vi "Main.vi"(11 "Module Admin":refnum<class "Delacor_lib_QMH_Module Admin.lvclass">) -> ()   [LabVIEW 2022 SP3, in "Event Manager.lvlib"]
doc: "This template is based from the Queued Message Handler design pattern and the Queued Message Handler Project Template that ships with LabVIEW 2014.\n\nThe main difference is that the Queue is private to this module and communication between modules is done via Broadcast and Request events.\n\nRequest events are wrapped via public API methods and are handled in the Event handler loop in this VI.\nAny module can register for Broadcast events sent by this module.\n\nThe Event Handling Loop generates messages based on user interface actions.\n\nThe Message Handling Loop processes messages generated by the Event Handling Loop, or by other messages. The messages are string values, so new messages can be added easily to the Message Cases case structure in the Message Handling Loop. Each message cluster can also provide an optional value for Message Data, which is a variant that can be converted to whatever message-specific data is required.\n____\nHAMPEL SOFTWARE ENGINEERING v2.6.0 (2023-12-19 10:54)"
uses:
  Event Manager.lvlib
  <vilib>/Delacor/Delacor QMH/Libraries/Module Admin_class/Delacor_lib_QMH_Module Admin.lvclass
  Libraries/hse-libraries/Source/hse-dqmh/Dynamic Requesters/Singleton/Status Updated Argument--cluster.ctl
  Libraries/hse-libraries/Source/hse-dqmh/Dynamic Requesters/Singleton/Error Reported Argument--cluster.ctl
  Libraries/hse-libraries/Source/hse-dqmh/Controls/System Message Argument--cluster.ctl
  Libraries/hse-libraries/Source/hse-dqmh/Controls/System Message Source.ctl
  Module Data--cluster.ctl
  Stop Argument--cluster.ctl
  <vilib>/Delacor/Delacor QMH/Libraries/Message Queue_class/Delacor_lib_QMH_Message Queue.lvclass/Delacor_lib_QMH_Message Queue.ctl
  <vilib>/Delacor/Delacor QMH/Libraries/Module Admin_class/Delacor_lib_QMH_Module Admin.lvclass/Delacor_lib_QMH_Module Admin.ctl
  Configure Argument--cluster.ctl
  Prepare Argument--cluster.ctl
  Set Modules Argument--cluster.ctl
  Set Modules (Reply Payload)--cluster.ctl
  <vilib>/Hampel Software Engineering/HSE Logger/LogRecord/LogRecord.lvclass/LogRecord.ctl
  Request UI Display Argument--cluster.ctl
  Libraries/hse-libraries/Source/hse-dqmh/Controls/Module Display Scenarios.ctl
  Request UI Display (Reply Payload)--cluster.ctl
  <vilib>/Utility/miscctls.llb/LVPointTypeDef.ctl
  <vilib>/Hampel Software Engineering/HSE Logger/LogRecord/LogRecord.lvclass
  <vilib>/Delacor/Delacor QMH/Libraries/Message Queue_class/Delacor_lib_QMH_Enqueue Message (Single).vi
  <vilib>/Delacor/Delacor QMH/Libraries/Module Admin_class/Delacor_lib_QMH_Get External Launch.vi
  <vilib>/Utility/error.llb/Error Cluster From Error Code.vi
  <vilib>/ErrorRing/Error Ring.xnode
  <vilib>/Delacor/Delacor QMH/Libraries/Message Queue_class/Delacor_lib_QMH_Message Queue.lvclass
  Libraries/hse-libraries/Source/hse-configuration/config-ini/config-ini.lvclass
  <vilib>/Hampel Software Engineering/HSE Logger/hse-logger.lvlib
  Libraries/hse-libraries/Source/hse-dqmh/hse-dqmh-dynamicrequesters.lvlib
  Libraries/hse-libraries/Source/hse-dqmh/hse-dqmh.lvlib
  Libraries/hse-libraries/Source/hse-misc/hse-misc.lvlib
panel:
  out "max rows":i32
  out "Status Bar":string
  in  "Event Log":i32(listbox)=-1
  out "error out":errorcluster
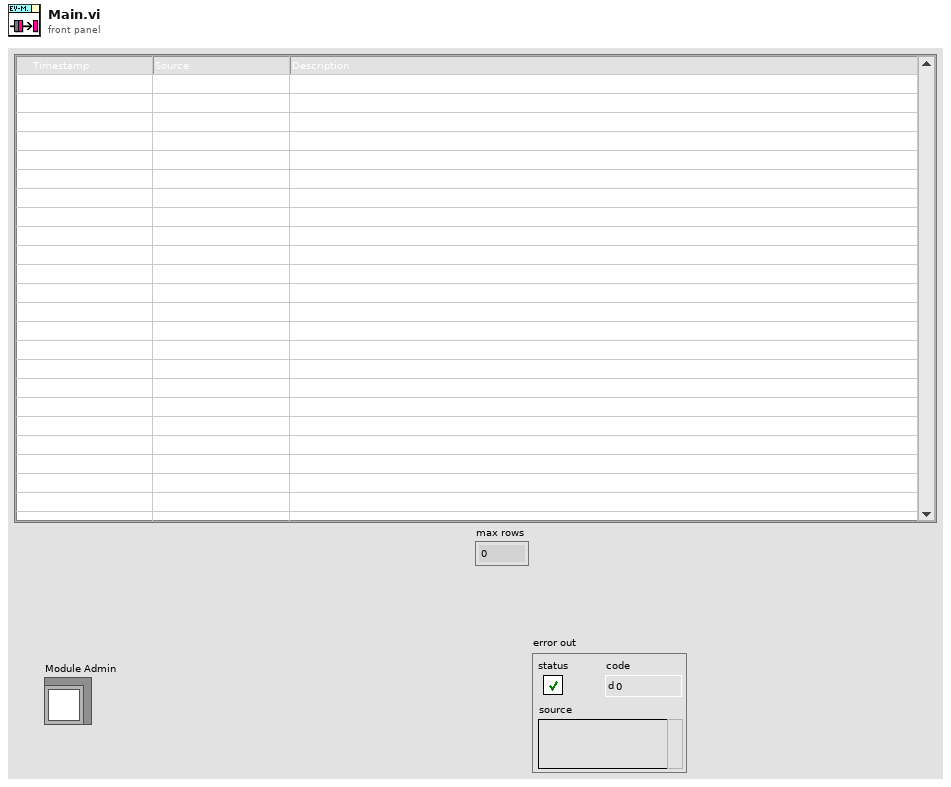
[diagram p1: front panel]
types:
  T1 = typedef "Event Manager.lvlib/Request Events--cluster.ctl" = cluster{"Stop Module":refnum<user-event>, "Show Panel":refnum<user-event>, "Hide Panel":refnum<user-event>, "Get Module Execution Status":refnum<user-event>, "Show Diagram":refnum<user-event>, "Configure":refnum<user-event>, "Prepare":refnum<user-event>, "Register for module events":refnum<user-event>, "Set Modules":refnum<user-event>, "Request UI Display":refnum<user-event>}
  T2 = typedef "Event Manager.lvlib/Module Data--cluster.ctl" = cluster{"Module Paths":path[]}
  T3 = enum32{"Invalid", "Standard", "Closed", "Hidden", "Minimized", "Maximized"}
  T4 = enum32{"invalid lock state", "Not Locked", "Locked (No Password)", "Password-protected"}
  T5 = typedef "Event Manager.lvlib/Stop Argument--cluster.ctl" = cluster{"Origin":string, "Exit via Stop Module Req?":bool, "Wait for Module to stop?":bool}
  T6 = typedef "Event Manager.lvlib/Configure Argument--cluster.ctl" = cluster{"Boolean":bool}
  T7 = typedef "Event Manager.lvlib/Prepare Argument--cluster.ctl" = cluster{"Boolean":bool}
  T8 = typedef "Event Manager.lvlib/Set Modules Argument--cluster.ctl" = cluster{"Module Paths":path[], "Wait Notifier":refnum<notifier>, "wait for reply":bool}
  T9 = typedef "Event Manager.lvlib/Request UI Display Argument--cluster.ctl" = cluster{"Scenario":T10, "Wait Notifier":refnum<notifier>, "wait for reply":bool}
  T10 = typedef "hse-dqmh.lvlib/Module Display Scenarios.ctl" = enum16{"Stand-Alone", "Managed"}
  T11 = typedef "LVPointTypeDef.ctl" = cluster{"Horizontal":i16, "Vertical":i16}
  T12 = typedef "Event Manager.lvlib/Request UI Display (Reply Payload)--cluster.ctl" = cluster{"Accept?":bool, "error":errorcluster}
  T13 = typedef "Event Manager.lvlib/Set Modules (Reply Payload)--cluster.ctl" = cluster{"Set Modules_error":errorcluster}
  T14 = typedef "LVRectTypeDef.ctl" = cluster{"Left":i16, "Top":i16, "Right":i16, "Bottom":i16}
  T15 = typedef "hse-logger.lvlib/LogLevel.ctl" = enum16{"DEBUG", "INFO", "WARNING", "ERROR", "CRITICAL"}
  T16 = typedef "hse-dqmh.lvlib/System Message Source.ctl" = enum16{"module", "application", "network"}
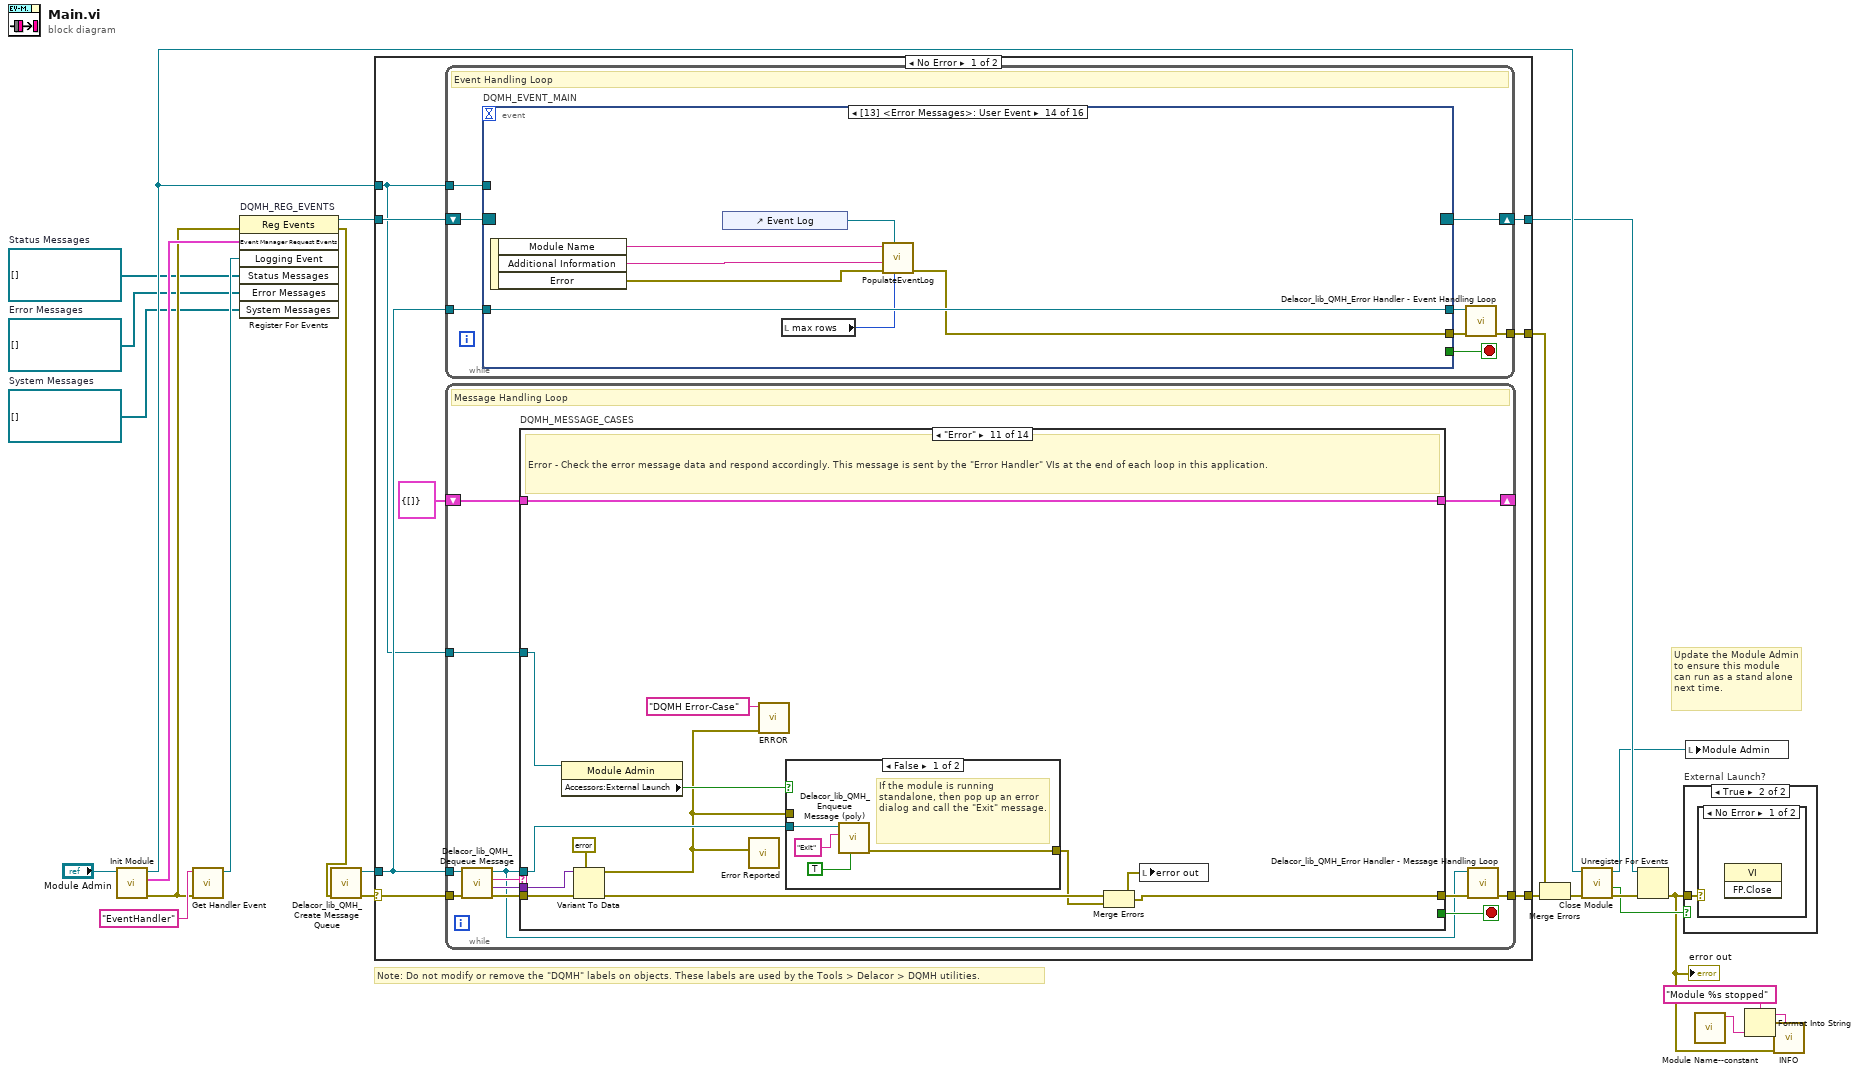
[diagram p0: block diagram]
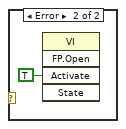
[diagram p3: hidden frame]
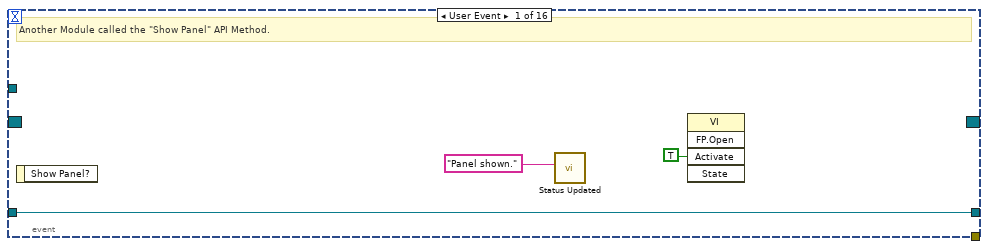
[diagram p4: hidden frame]
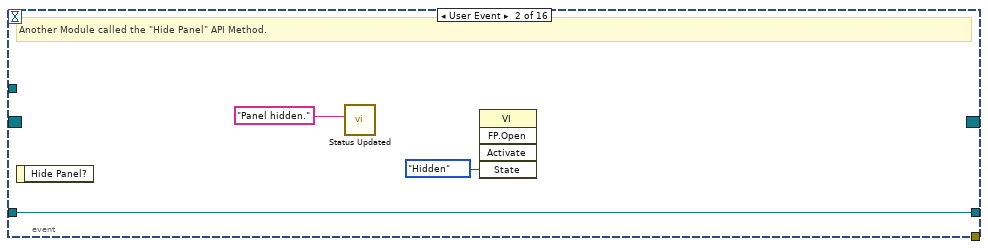
[diagram p5: hidden frame]
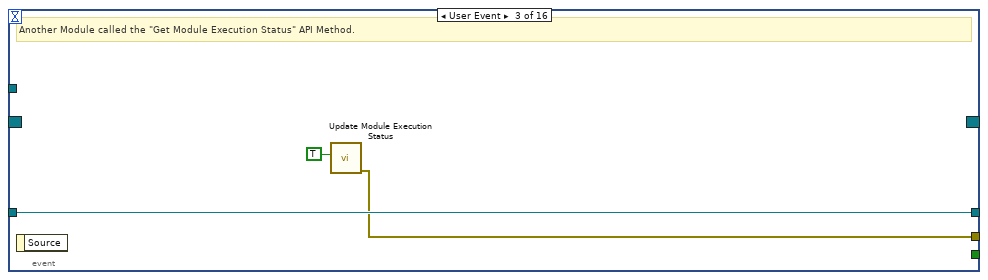
[diagram p6: hidden frame]
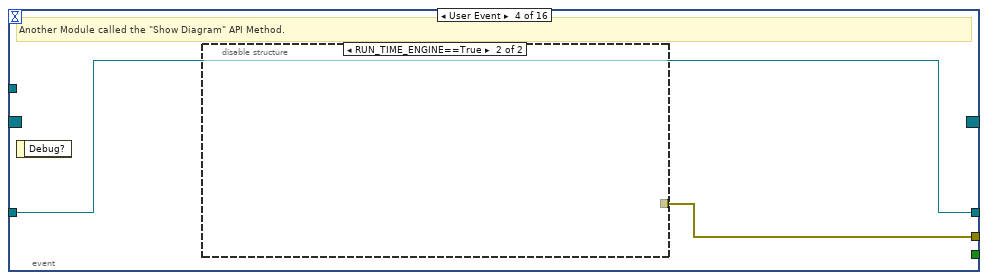
[diagram p7: hidden frame]
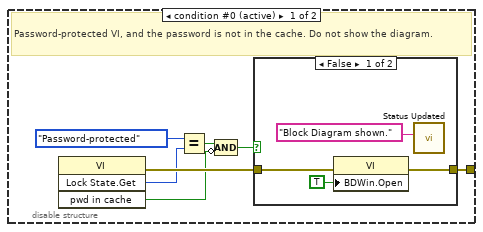
[diagram p8: hidden frame]
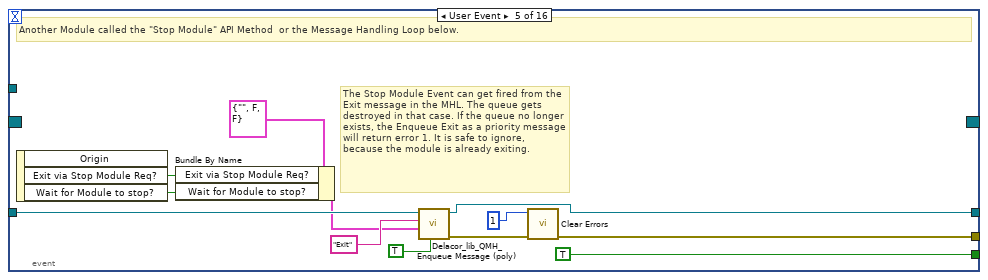
[diagram p10: hidden frame]
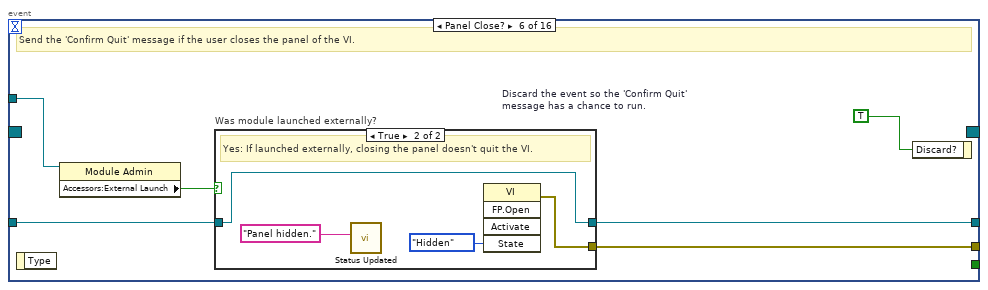
[diagram p11: hidden frame]
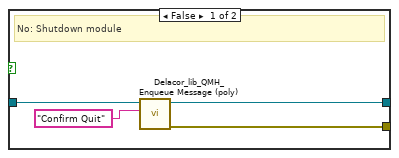
[diagram p12: hidden frame]
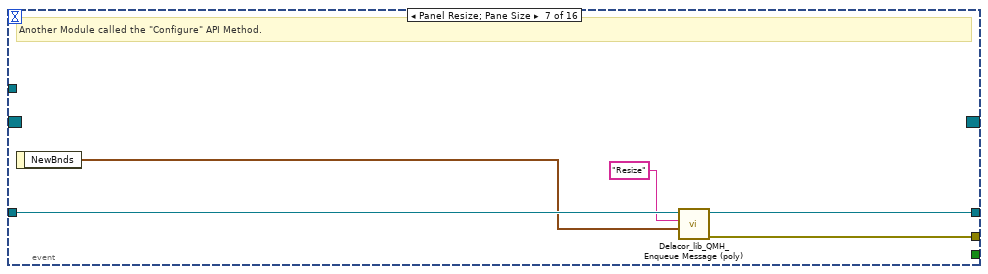
[diagram p13: hidden frame]
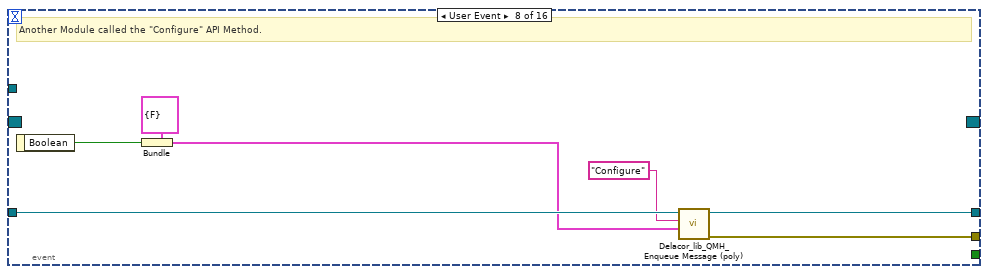
[diagram p14: hidden frame]
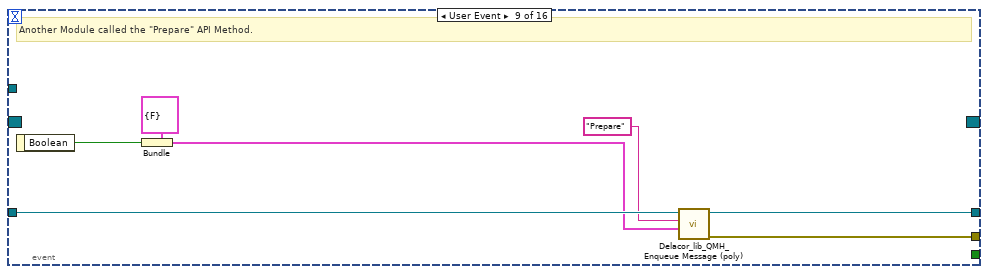
[diagram p15: hidden frame]
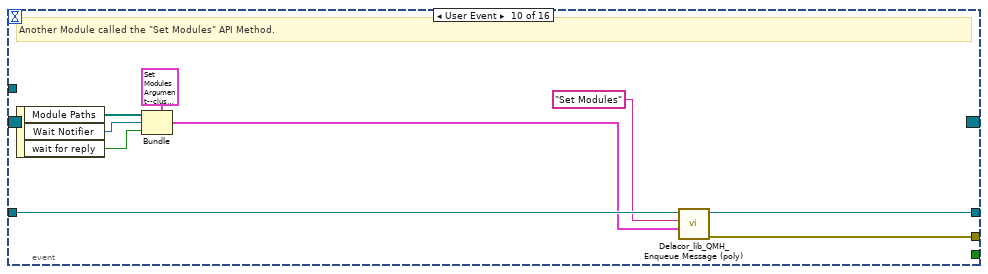
[diagram p16: hidden frame]
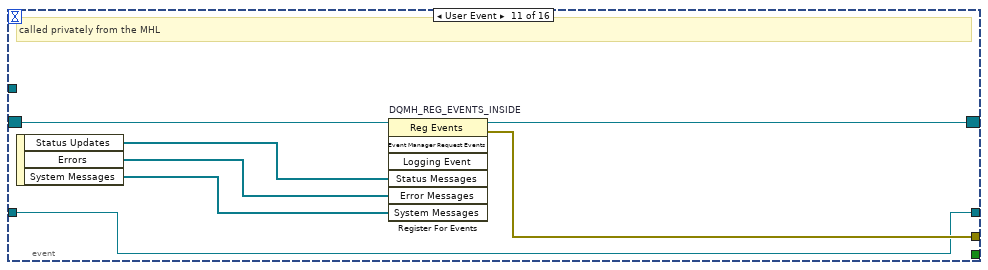
[diagram p17: hidden frame]
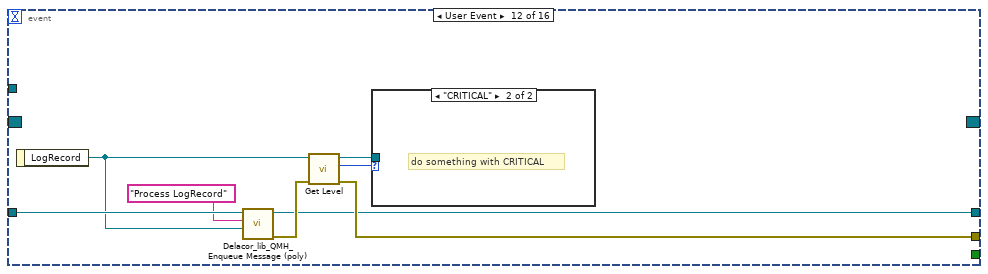
[diagram p18: hidden frame]
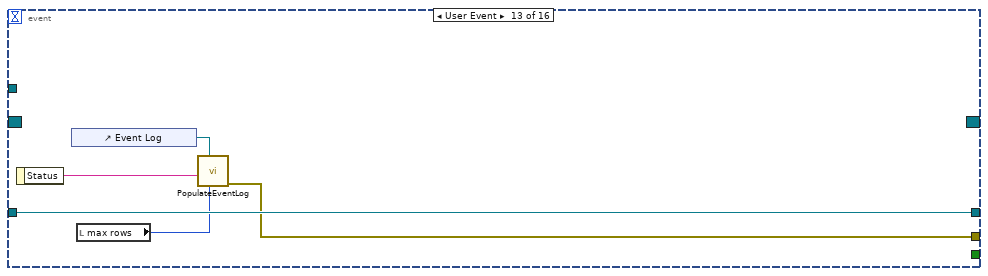
[diagram p20: hidden frame]
diagram:
  w1 = refnum<user-event>[] []  # System Messages
  w2 = refnum<user-event>[] []  # Error Messages
  w3 = refnum<user-event>[] []  # Status Messages
  # "Note: Do not modify or remove the \"DQMH\" labels on objects. These labels are used by the Tools > Delacor > DQMH utilities."
  # "Update the Module Admin to ensure this module can run as a stand alone next time."
  n1 = call "Init Module.vi"("Singleton Module Admin in"="Module Admin") -> ("error out"=w5:errorcluster, "Event Manager Request Events"=w20:T1, "Singleton Module Admin out"=w24:refnum<class "Delacor_lib_QMH_Module Admin.lvclass">)  [unwired: 8 in]
  n2 = call <vilib>:"Get Handler Event.vi"("error in"=w5, "Name"="EventHandler") -> ("Logging Event"=w11:refnum<user-event>)  [unwired: 8 in, 1 out]
  n3 = register-events "DQMH_REG_EVENTS"(error in=w5, w20, w11, w3, w2, w1) -> (reference out=w21:refnum<event-registration>, error out=w4:errorcluster)  [unwired: 1 in]
  n4 = call <vilib>:"Delacor_lib_QMH_Create Message Queue.vi"("error in"=w4) -> ("error out"=w12:errorcluster, "Message Queue"=w19:refnum<class "Delacor_lib_QMH_Message Queue.lvclass">)  [unwired: 9 in]
  n5 = case shown="No Error" w12 {
    selector: w12 -> [w26 w372]
    tunnel: [w32 w372] -> w23
    tunnel: [w31 w377] -> w22
    tunnel: w21 -> [w29 w377]
    tunnel: w19 -> [w28 w369]
    tunnel: [w27 _] -> w15
    tunnel: w24 -> [w25 w373]
    frame No Error {
      n6 = while {
        tunnel: w28 -> [w40]
        shift-right: [w38] -> w31
        shift-left: w29 -> [w39]
        tunnel: [w34] -> w27
        tunnel: w25 -> [w33]
        stop <- w36 stop-if-true
        # "Event Handling Loop"
        n7 = event "DQMH_EVENT_MAIN" shown="[13] <Error Messages>: User Event" {
          selector: w39 -> [_ _ _ _ _ _ _ _ _ _ w124 _ _ _ _ _]
          dyn-events: [_ _ _ _ _ _ _ _ _ _ w123 _ _ _ _ _] -> w38
          timeout: _ -> [_ _ _ _ _ _ _ _ _ _ _ _ _ _ _ _]
          tunnel: [_ _ _ _ TRUE ("Discard?") _ _ _ _ _ _ _ _ _ _ _] -> w36
          tunnel: w40 -> [w43 w46 w49 w50 w73 w80 w94 w101 w108 w117 w118 w130 w137 w144 w155 w165]
          tunnel: [_ _ w48 w51 w68 w79 w91 w95 w102 w109 w119 w132 w134 w142 w156 w157] -> w37
          tunnel: [w43 w46 w49 w50 w72 w78 w93 w100 w107 w116 w118 w129 w137 w144 w155 w164] -> w35
          tunnel: w33 -> [_ _ _ _ _ w77 _ _ _ _ _ _ _ _ _ _]
          event User Event {
            # "Another Module called the \"Show Panel\" API Method."
            n8 = event-data() -> ()  [unwired: 1 in, 1 out]
            n9 = call "Status Updated.vi"("Status"="Panel shown." ("format string")) -> ()  [unwired: 10 in, 1 out]
            n10 = invoke class="VI" method="FP.Open"("Activate"=TRUE ("Activate?")) -> ()  [unwired: 4 in, 5 out]
          }
          event User Event {
            # "Another Module called the \"Hide Panel\" API Method."
            n11 = event-data() -> ()  [unwired: 1 in, 1 out]
            n12 = call "Status Updated.vi"("Status"="Panel hidden." ("format string")) -> ()  [unwired: 10 in, 1 out]
            n13 = invoke class="VI" method="FP.Open"("State"=T3."Hidden") -> ()  [unwired: 4 in, 5 out]
          }
          event User Event {
            # "Another Module called the \"Get Module Execution Status\" API Method."
            n14 = event-data() -> ()  [unwired: 1 in, 1 out]
            n15 = call "Update Module Execution Status.vi"("Running?"=TRUE) -> ("error out"=w48:errorcluster)  [unwired: 10 in]
          }
          event User Event {
            # "Another Module called the \"Show Diagram\" API Method."
            n16 = event-data() -> ()  [unwired: 1 in, 1 out]
            n17 = disable-structure shown="RUN_TIME_ENGINE==True" {
              disable-tunnel: [w58 _] -> w51
              frame condition #0 (active) {
                # "Password-protected VI, and the password is not in the cache. Do not show the diagram."
                n18 = invoke class="VI" method="Lock State.Get"() -> (error out=w57:errorcluster, "Get Lock State"=w56:T4, "pwd in cache"=w53:bool)  [unwired: 4 in, 1 out]
                n19 = Equal?(x=T4."Password-protected", y=w56) -> (x = y?=w54:bool)
                n20 = Compound Arithmetic op=AND(w54, invert w53) -> (w52:bool)
                n21 = case shown="False" w52 {
                  tunnel: [w61 w63] -> w58
                  tunnel: w57 -> [w59 w63]
                  frame False {
                    n22 = property class="VI"(error in=w59, "BDWin.Open"=TRUE ("Block Diagram Window:Open")) -> (error out=w61:errorcluster)  [unwired: 1 in, 1 out]
                    n23 = call "Status Updated.vi"("Status"="Block Diagram shown." ("format string")) -> ()  [unwired: 10 in, 1 out]
                  }
                  frame True {
                    # "Password-protected VI, and the password is not in the cache. Do not show the diagram."
                  }
                }
              }
              frame condition #1 {
              }
            }
          }
          event User Event {
            # "The Stop Module Event can get fired from the Exit message in the MHL. The queue gets destroyed in that case. If the queue no longer exists, the Enqueue Exit as a priority message will return error 1. It is safe to ignore, because the module is already exiting."
            # "Another Module called the \"Stop Module\" API Method  or the Message Handling Loop below."
            n24 = event-data() -> ("Exit via Stop Module Req?"=w66:bool, "Wait for Module to stop?"=w65:bool)  [unwired: 1 in, 1 out]
            n25 = Bundle By Name(cluster=T5 {"Origin"="", "Exit via Stop Module Req?"=FALSE, "Wait for Module to stop?"=FALSE} ("Stop Argument"), "Exit via Stop Module Req?"=w66, "Wait for Module to stop?"=w65) -> (w64:T5)
            n26 = call-poly <vilib>:"Delacor_lib_QMH_Enqueue Message (poly).vi"("Priority Message? (F)"=TRUE, "Message Data"=w64, "Message"="Exit", "Message Queue in"=w73) -> ("error out"=w69:errorcluster, "Message Queue out"=w72:refnum<class "Delacor_lib_QMH_Message Queue.lvclass">)  [unwired: 6 in]
            n27 = call <vilib>:"Clear Errors.vi"("error in (no error)"=w69, "specific error code to clear (0: all)"=1) -> ("error out"=w68:errorcluster)  [unwired: 4 in, 1 out]
          }
          event Panel Close? {
            w81 = TRUE  # Discard the event so the 'Confirm Quit' message has a chance to run.
            # "Send the 'Confirm Quit' message if the user closes the panel of the VI."
            n28 = event-data() -> ()  [unwired: 1 in, 1 out]
            n29 = property class="Module Admin"(reference=w77) -> ("Accessors:External Launch"=w76:bool)  [unwired: 1 in, 2 out]
            n30 = case "Was module launched externally?" shown="True" w76 {
              tunnel: w80 -> [w85 w87]
              tunnel: [w84 w86] -> w79
              tunnel: [w83 w87] -> w78
              frame False {
                # "No: Shutdown module"
                n31 = call-poly <vilib>:"Delacor_lib_QMH_Enqueue Message (poly).vi"("Message"="Confirm Quit", "Message Queue in"=w85) -> ("error out"=w84:errorcluster, "Message Queue out"=w83:refnum<class "Delacor_lib_QMH_Message Queue.lvclass">)  [unwired: 8 in]
              }
              frame True {
                # "Yes: If launched externally, closing the panel doesn't quit the VI."
                n32 = call "Status Updated.vi"("Status"="Panel hidden." ("format string")) -> ()  [unwired: 10 in, 1 out]
                n33 = invoke class="VI" method="FP.Open"("State"=T3."Hidden") -> (error out=w86:errorcluster)  [unwired: 4 in, 4 out]
              }
            }
            n34 = event-data("Discard?"=w81) -> ()  [unwired: 1 in, 1 out]
          }
          event Panel Resize; Pane Size {
            # "Another Module called the \"Configure\" API Method."
            n35 = event-data() -> ("NewBnds"=w90:T14)  [unwired: 1 in]
            n36 = call-poly <vilib>:"Delacor_lib_QMH_Enqueue Message (poly).vi"("Message Data"=w90, "Message"="Resize", "Message Queue in"=w94) -> ("error out"=w91:errorcluster, "Message Queue out"=w93:refnum<class "Delacor_lib_QMH_Message Queue.lvclass">)  [unwired: 7 in]
          }
          event User Event {
            # "Another Module called the \"Configure\" API Method."
            n37 = event-data() -> ("Boolean"=w96:bool)  [unwired: 1 in]
            n38 = Bundle(cluster=T6 {"Boolean"=FALSE} ("Configure Argument"), "Boolean"=w96) -> (w97:T6)
            n39 = call-poly <vilib>:"Delacor_lib_QMH_Enqueue Message (poly).vi"("Message Data"=w97, "Message"="Configure", "Message Queue in"=w101) -> ("error out"=w95:errorcluster, "Message Queue out"=w100:refnum<class "Delacor_lib_QMH_Message Queue.lvclass">)  [unwired: 7 in]
          }
          event User Event {
            # "Another Module called the \"Prepare\" API Method."
            n40 = event-data() -> ("Boolean"=w103:bool)  [unwired: 1 in]
            n41 = Bundle(cluster=T7 {"Boolean"=FALSE} ("Prepare Argument"), "Boolean"=w103) -> (w104:T7)
            n42 = call-poly <vilib>:"Delacor_lib_QMH_Enqueue Message (poly).vi"("Message Data"=w104, "Message"="Prepare", "Message Queue in"=w108) -> ("error out"=w102:errorcluster, "Message Queue out"=w107:refnum<class "Delacor_lib_QMH_Message Queue.lvclass">)  [unwired: 7 in]
          }
          event User Event {
            # "Another Module called the \"Set Modules\" API Method."
            n43 = event-data() -> ("Module Paths"=w112:path[], "Wait Notifier"=w111:refnum<notifier>, "wait for reply"=w110:bool)  [unwired: 1 in]
            n44 = Bundle(cluster=T8 {"Module Paths"=[path "Modules/Dummie"], "Wait Notifier"=refnum, "wait for reply"=FALSE} ("Set Modules Argument"), "Module Paths"=w112, "Wait Notifier"=w111, "wait for reply"=w110) -> (w113:T8)
            n45 = call-poly <vilib>:"Delacor_lib_QMH_Enqueue Message (poly).vi"("Message Data"=w113, "Message"="Set Modules", "Message Queue in"=w117) -> ("error out"=w109:errorcluster, "Message Queue out"=w116:refnum<class "Delacor_lib_QMH_Message Queue.lvclass">)  [unwired: 7 in]
          }
          event User Event {
            # "called privately from the MHL"
            n46 = event-data() -> ("Status Updates"=w122:refnum<user-event>[], "Errors"=w121:refnum<user-event>[], "System Messages"=w120:refnum<user-event>[])  [unwired: 1 in]
            n47 = register-events "DQMH_REG_EVENTS_INSIDE"(reference=w124, w122, w121, w120) -> (reference out=w123:refnum<event-registration>, error out=w119:errorcluster)  [unwired: 3 in]
          }
          event User Event {
            n48 = event-data() -> ("LogRecord"=w127:refnum<class "LogRecord.lvclass">)  [unwired: 1 in]
            n49 = call-poly <vilib>:"Delacor_lib_QMH_Enqueue Message (poly).vi"("Message Data"=w127, "Message"="Process LogRecord", "Message Queue in"=w130) -> ("error out"=w131:errorcluster, "Message Queue out"=w129:refnum<class "Delacor_lib_QMH_Message Queue.lvclass">)  [unwired: 7 in]
            n50 = call <vilib>:"Get Level.vi"("error in"=w131, "LogRecord in"=w127) -> ("error out"=w132:errorcluster, "Level"=w126:T15, "LogRecord out"=w125:refnum<class "LogRecord.lvclass">)  [unwired: 7 in]
            n51 = case shown="\"CRITICAL\"" w126 {
              tunnel: w125 -> [_ _]
              frame Default {
              }
              frame "CRITICAL" {
                # "do something with CRITICAL"
              }
            }
          }
          event User Event {
            n52 = event-data() -> ("Status"=w136:string)  [unwired: 1 in]
            n53 = control-ref of="Event Log"() -> (w135:refnum<vi>)
            n54 = local read "max rows"() -> (w133:i32)
            n55 = call "PopulateEventLog.vi"("max rows"=w133, "Listbox"=w135, "Additional Information"=w136) -> ("error out"=w134:errorcluster)  [unwired: 6 in, 2 out]
          }
          event User Event {
            n56 = event-data() -> ("Module Name"=w139:string, "Additional Information"=w141:string, "Error"=w140:errorcluster)  [unwired: 1 in]
            n57 = control-ref of="Event Log"() -> (w143:refnum<vi>)
            n58 = local read "max rows"() -> (w138:i32)
            n59 = call "PopulateEventLog.vi"("max rows"=w138, "Listbox"=w143, "error in"=w140, "Additional Information"=w141, "Module Name"=w139) -> ("error out"=w142:errorcluster)  [unwired: 4 in, 2 out]
          }
          event User Event {
            n60 = event-data() -> ("Identifier"=w150:string, "Payload"=w149:variant, "Sys. Msg. Source"=w148:T16, "Sys. Msg. Origin"=w147:string)  [unwired: 1 in]
            n61 = call "Interpret System Message Event Data.vi"("Sys. Msg. Origin"=w147, "Sys. Msg. Source"=w148, "Payload"=w149, "Identifier"=w150) -> ("error out"=w146:errorcluster, "Additional Info"=w152:string, "Module ID"=w151:i32, "Module Name"=w154:string)  [unwired: 4 in]
            n62 = control-ref of="Event Log"() -> (w153:refnum<vi>)
            n63 = local read "max rows"() -> (w145:i32)
            n64 = call "PopulateEventLog.vi"("max rows"=w145, "Listbox"=w153, "error in"=w146, "Additional Information"=w152, "Module ID"=w151, "Module Name"=w154) -> ("error out"=w156:errorcluster)  [unwired: 3 in, 2 out]
          }
          event User Event {
            # "Another Module called the \"Request UI Display\" API Method."
            n65 = event-data() -> ("Scenario"=w160:T10, "Wait Notifier"=w159:refnum<notifier>, "wait for reply"=w158:bool)  [unwired: 1 in]
            n66 = Bundle(cluster=T9 {"Scenario"=enum."Stand-Alone", "Wait Notifier"=refnum, "wait for reply"=FALSE} ("Request UI Display Argument"), "Scenario"=w160, "Wait Notifier"=w159, "wait for reply"=w158) -> (w161:T9)
            n67 = call-poly <vilib>:"Delacor_lib_QMH_Enqueue Message (poly).vi"("Message Data"=w161, "Message"="Request UI Display", "Message Queue in"=w165) -> ("error out"=w157:errorcluster, "Message Queue out"=w164:refnum<class "Delacor_lib_QMH_Message Queue.lvclass">)  [unwired: 7 in]
          }
        }
        n68 = call-dynamic "Delacor_lib_QMH_Error Handler - Event Handling Loop.vi"("error in"=w37, "Message Queue in"=w35) -> ("dup error in"=w34:errorcluster)  [unwired: 8 in, 1 out]
      }
      n69 = while {
        tunnel: w28 -> [w169]
        shift-right: [w175] -> _
        shift-left: T2 {"Module Paths"=[]} ("Data Cluster") -> [w176]
        tunnel: w26 -> [w173]
        tunnel: [w167] -> w32
        tunnel: w25 -> [w166]
        stop <- w174 stop-if-true
        # "Message Handling Loop"
        n70 = call-dynamic "Delacor_lib_QMH_Dequeue Message.vi"("error in"=w173, "Message Queue in"=w169) -> ("error out"=w172:errorcluster, "Message Data"=w170:variant, "Message"=w171:string, "Message Queue out"=w168:refnum<class "Delacor_lib_QMH_Message Queue.lvclass">)  [unwired: 6 in]
        n71 = case "DQMH_MESSAGE_CASES" shown="\"Error\"" w171 {
          selector: w171 -> [_ _ _ _ _ _ _ _ _ _ _ _ _ w358]
          tunnel: w168 -> [_ _ _ _ _ _ _ _ _ _ w324 w337 w354 _]
          tunnel: w172 -> [w192 w207 w212 w231 w236 w251 w267 w281 w314 w318 w330 w341 w356 _]
          tunnel: [w187 w205 w222 w230 w235 w244 w265 w282 w308 w316 w321 w339 w351 w359] -> w177
          tunnel: w176 -> [w191 w206 w223 w234 w239 w250 w266 w272 w300 w317 w329 w340 w342 w360]
          tunnel: [w191 w206 w223 w234 w239 w250 w266 w271 w300 w317 w329 w340 w342 w360] -> w175
          tunnel: [_ _ _ _ _ _ _ _ _ _ _ _ w353 _] -> w174
          tunnel: w170 -> [_ _ _ _ _ w248 _ w280 w313 _ w328 _ w350 _]
          tunnel: w166 -> [w193 _ _ _ _ _ _ _ _ _ w323 _ w343 _]
          frame "Initialize" {
            w182 = string[][] []  # Item Names
            # "Initialize - Any operation that needs to be done before the module can receive messages. Synchronize Caller Events.vi will inform Start Module.vi that the module has launched and is ready to receive messages. Module Did Init.vi will broadcast that the module initialized."
            n72 = call "Synchronize Caller Events.vi"("error in (no error)"=w192, "Singleton Module Admin in"=w193) -> ("error out"=w189:errorcluster, "Singleton Module Admin out"=w188:refnum<class "Delacor_lib_QMH_Module Admin.lvclass">)  [unwired: 8 in]
            n73 = disable-structure shown="Default" {
              disable-tunnel: w188 -> [w195 _]
              frame condition #0 (active) {
                # "(Embedded) UI available"
                n74 = property class="Module Admin"(reference=w195) -> ("Accessors:External Launch"=w199:bool)  [unwired: 1 in, 2 out]
                n75 = property on="Pane" class="Pane"("Origin"=T11 {"Horizontal"=0, "Vertical"=0}) -> ()  [unwired: 2 in, 2 out]
                n76 = Select(t=T3."Hidden" ("State"), s=w199, f=T3."Standard" ("State")) -> (s? t:f=w196:T3)
                n77 = call "Module Name--constant.vi"() -> ("Module Name"=w204:string)  [unwired: 11 in]
                n78 = property class="VI"("Front Panel.Title"=w204) -> (reference out=w202:refnum<vi>, error out=w203:errorcluster)  [unwired: 2 in]
                n79 = invoke class="VI" method="FP.Open"(reference=w202, error in=w203, "State"=w196) -> (reference out=w201:refnum<vi>, error out=w200:errorcluster)  [unwired: 2 in, 3 out]
                n80 = invoke class="VI" method="FP.Center"(reference=w201, error in=w200) -> ()  [unwired: 1 in, 3 out]
              }
              frame condition #1 {
                # "No embedded UI available"
              }
            }
            n81 = control-ref of="Event Log"() -> (w183:refnum<vi>)
            n82 = call "Module Name--constant.vi"() -> ("Module Name"=w186:string)  [unwired: 11 in]
            n83 = property class="MCListbox (strict)"(reference=w183, "ItemNames"=w182) -> (reference out=w178:refnum<vi>)  [unwired: 1 in, 1 out]
            n84 = call "Module Did Init.vi"("error in (no error)"=w189, "Initialized?"=TRUE, "Origin"=w186) -> ("error out"=w180:errorcluster)  [unwired: 8 in]
            n85 = control-ref of="This VI"() -> (w181:refnum<vi>)
            n86 = call "Tidy Up MCLB UI.vi"("error in (no error)"=w180, "Event Log"=w178, "VI in"=w181) -> ("error out"=w179:errorcluster)  [unwired: 8 in]
            n87 = Format Into String(format string="Module %s initialised", w186) -> (resulting string=w185:string)  [unwired: 2 in, 1 out]
            n88 = call <vilib>:"INFO.vi"("Message"=w185, "error in"=w179) -> ("error out"=w187:errorcluster)  [unwired: 9 in]
          }
          frame "--- Setup ---" {
            # "Separator -- The following cases handle messages specific to this Module."
            n89 = Merge Errors(w207) -> (w205:errorcluster)
          }
          frame "Configure" {
            # "Triggers the auto-configuration of the module."
            n90 = call "Module Name--constant.vi"() -> ("Module Name"=w214:string)  [unwired: 11 in]
            n91 = call "Create Module Config.vi"("error in"=w212, "DQMH Module Name"=w214) -> ("error out"=w216:errorcluster, "config-ini out"=w215:refnum<class "config-ini.lvclass">)  [unwired: 8 in]
            n92 = call-dynamic "Read Integer.vi"("Section"="global", "error in"=w216, "Key"="max rows", "config-base in"=w215) -> ("error out"=w213:errorcluster, "Value"=w209:i64)  [unwired: 5 in, 1 out]
            n93 = To Long Integer(number=w209) -> (32bit integer=w208:i32)
            n94 = case shown="No Error" w213 {
              selector: w213 -> [w225 w228]
              tunnel: [w225 errorcluster {"status"=FALSE, "code"=0, "source"=""} ("error IO")] -> w211
              tunnel: [w224 100 ("max rows")] -> w210
              tunnel: w208 -> [w224 _]
              frame No Error {
              }
              frame Error {
                n95 = call <vilib>:"WARNING.vi"("Message"="Could not read key \"max_rows\" in  config \"Event Manager.ini\". Using default value of 100 rows.", "error in"=w228) -> ()  [unwired: 9 in, 1 out]
              }
            }
            "max rows" <- w210
            n96 = call "Module Name--constant.vi"() -> ("Module Name"=w221:string)  [unwired: 11 in]
            n97 = Format Into String(format string="Module %s configured.", w221) -> (resulting string=w219:string)  [unwired: 2 in, 1 out]
            n98 = call <vilib>:"INFO.vi"("Message"=w219, "error in"=w211) -> ("error out"=w222:errorcluster)  [unwired: 9 in]
          }
          frame "Prepare" {
            # "Prepares the front panel for display"
            n99 = control-ref of="Event Log"() -> (w233:refnum<vi>)
            n100 = control-ref of="This VI"() -> (w232:refnum<vi>)
            n101 = call "Tidy Up MCLB UI.vi"("error in (no error)"=w231, "Event Log"=w233, "VI in"=w232) -> ("error out"=w230:errorcluster)  [unwired: 8 in]
          }
          frame "Resize" {
            n102 = control-ref of="Event Log"() -> (w238:refnum<vi>)
            n103 = control-ref of="This VI"() -> (w237:refnum<vi>)
            n104 = call "Tidy Up MCLB UI.vi"("error in (no error)"=w236, "Event Log"=w238, "VI in"=w237) -> ("error out"=w235:errorcluster)  [unwired: 8 in]
          }
          frame "Request UI Display" {
            # "Requests the module to display its UI as specified in <b>Scenario</b>:\n\"managed\" => in the UI Manager's subpanel\n\"stand-alone\" => as a separate window"
            n105 = Variant To Data(error in=w251, type=T9 {"Scenario"=enum."Stand-Alone", "Wait Notifier"=refnum, "wait for reply"=FALSE} ("Request UI Display Argument"), Variant=w248) -> (data=w243:T9, error out=w249:errorcluster)
            n106 = Unbundle By Name(w243) -> ("Scenario"=w240:T10, "Wait Notifier"=w246:refnum<notifier>, "wait for reply"=w245:bool)
            n107 = control-ref of="This VI"() -> (w242:refnum<vi>)
            n108 = case shown="\"Stand-Alone\", Default" w240 {
              tunnel: w242 -> [w253 w259]
              tunnel: [w252 w255] -> w241
              frame "Stand-Alone", Default {
                n109 = invoke class="VI" method="FP.Open"(reference=w253, "Activate"=TRUE ("Activate?")) -> (error out=w252:errorcluster)  [unwired: 3 in, 4 out]
              }
              frame "Managed" {
                n110 = call "DQMH System Message - Ready for Display.vi"("Main VI Reference"=w259) -> ("Payload"=w256:variant, "Identifier"=w257:string, "Source"=w258:T16)  [unwired: 8 in]
                n111 = call "System Message.vi"("Sys. Msg. Source"=w258, "Payload"=w256, "Identifier"=w257) -> ("error out"=w255:errorcluster)  [unwired: 8 in]
              }
            }
            n112 = case shown="True" w245 {
              tunnel: w246 -> [_ w264]
              tunnel: w241 -> [_ w260]
              frame False {
              }
              frame True {
                n113 = Bundle By Name(cluster=T12 {"Accept?"=FALSE, "error"={"status"=FALSE, "code"=0, "source"=""}} ("Request UI Display (Reply Payload)"), "Accept?"=TRUE, "error"=w260) -> (w262:T12)
                n114 = Send Notification(notification=w262, notifier=w264) -> ()  [unwired: 1 in, 2 out]
              }
            }
            n115 = Merge Errors(w249, w241) -> (w244:errorcluster)
          }
          frame "--- Module Specific ---" {
            # "Separator -- The following cases handle messages specific to this Module."
            n116 = Merge Errors(w267) -> (w265:errorcluster)
          }
          frame "Set Modules" {
            # "Tells the EVH module which modules are loaded so EVH can register for their broadcasts."
            n117 = Variant To Data(error in=w281, type=T8 {"Module Paths"=[path "Modules/Dummie"], "Wait Notifier"=refnum, "wait for reply"=FALSE} ("Set Modules Argument"), Variant=w280) -> (data=w278:T8, error out=w283:errorcluster)
            n118 = Unbundle By Name(w272) -> ("Module Paths"=w269:path[])
            n119 = Unbundle By Name(w278) -> ("Module Paths"=w273:path[], "Wait Notifier"=w277:refnum<notifier>, "wait for reply"=w276:bool)
            n120 = control-ref of="This Application"() -> (w268:refnum<vi>)
            n121 = call "Register Modules in Event Manager--helper.vi"("Application in"=w268, "error in (no error)"=w283, "New Modules"=w273, "Modules IN"=w269) -> ("error out"=w282:errorcluster, "Modules OUT"=w270:path[])  [unwired: 6 in]
            n122 = Bundle By Name(cluster=T13 {"Set Modules_error"={"status"=FALSE, "code"=0, "source"=""}} ("Set Modules (Reply Payload)"), "Set Modules_error"=w282) -> (w275:T13)
            n123 = Bundle By Name(cluster=w272, "Module Paths"=w270) -> (w271:T2)
            n124 = case shown="True" w276 {
              tunnel: w277 -> [_ w285]
              tunnel: w275 -> [_ w284]
              frame False {
              }
              frame True {
                n125 = Send Notification(notification=w284, notifier=w285) -> ()  [unwired: 1 in, 2 out]
              }
            }
          }
          frame "Process LogRecord" {
            # "make all level values the same \nlength for visual alignment"
            n126 = Variant To Data(error in=w314, type=refnum<class "LogRecord.lvclass"> refnum ("LogRecord"), Variant=w313) -> (data=w298:refnum<class "LogRecord.lvclass">, error out=w295:errorcluster)
            n127 = call <vilib>:"Get Callchain.vi"("error in"=w295, "LogRecord in"=w298) -> ("error out"=w296:errorcluster, "Callchain"=w294:string, "LogRecord out"=w297:refnum<class "LogRecord.lvclass">)  [unwired: 7 in]
            n128 = call <vilib>:"Get Level.vi"("error in"=w296, "LogRecord in"=w297) -> ("error out"=w291:errorcluster, "Level"=w303:T15, "LogRecord out"=w292:refnum<class "LogRecord.lvclass">)  [unwired: 7 in]
            n129 = Format Into String(format string="%s", w303) -> (resulting string=w306:string)  [unwired: 2 in, 1 out]
            n130 = call "String_PadWithCharacters.vi"("char (ASCII)"=u8 32, "length"=8, "str in"=w306) -> ("str (padded)"=w302:string)  [unwired: 8 in]
            n131 = call <vilib>:"Get ISO Time.vi"("error in"=w291, "LogRecord in"=w292) -> ("error out"=w289:errorcluster, "ISO Time"=w287:string, "LogRecord out"=w290:refnum<class "LogRecord.lvclass">)  [unwired: 7 in]
            n132 = call <vilib>:"Get Message.vi"("error in"=w289, "LogRecord in"=w290) -> ("error out"=w310:errorcluster, "Message"=w288:string, "LogRecord out"=w311:refnum<class "LogRecord.lvclass">)  [unwired: 7 in]
            n133 = call <vilib>:"Get Error.vi"("error in"=w310, "LogRecord in"=w311) -> ("error out"=w315:errorcluster, "Error"=w299:errorcluster)  [unwired: 7 in, 1 out]
            n134 = control-ref of="Event Log"() -> (w301:refnum<vi>)
            n135 = local read "max rows"() -> (w286:i32)
            n136 = Format Into String(format string="%s - %s - %s", error in=w315, w302, w287, w288) -> (resulting string=w293:string, error out=w308:errorcluster)  [unwired: 1 in]
            n137 = call "PopulateEventLog.vi"("max rows"=w286, "Listbox"=w301, "error in"=w299, "Additional Information"=w293, "Module Name"=w294) -> ()  [unwired: 4 in, 3 out]
          }
          frame "--- Exit and Error Handling---" {
            # "Separator - The following cases handle errors and exit messages."
            n138 = Merge Errors(w318) -> (w316:errorcluster)
          }
          frame "Error" {
            # "Error - Check the error message data and respond accordingly. This message is sent by the \"Error Handler\" VIs at the end of each loop in this application."
            n139 = property class="Module Admin"(reference=w323) -> ("Accessors:External Launch"=w322:bool)  [unwired: 1 in, 2 out]
            n140 = Variant To Data(error in=w330, type=errorcluster {"status"=FALSE, "code"=0, "source"=""} ("error constant"), Variant=w328) -> (data=w320:errorcluster, error out=w326:errorcluster)
            n141 = call "Error Reported.vi"("Error"=w320) -> ()  [unwired: 10 in, 1 out]
            n142 = call <vilib>:"ERROR.vi"("Message"="DQMH Error-Case", "error in"=w320) -> ()  [unwired: 9 in, 1 out]
            n143 = case shown="False" w322 {
              tunnel: [w334 _] -> w325
              tunnel: w324 -> [w333 _]
              tunnel: w320 -> [_ _]
              frame False {
                # "If the module is running standalone, then pop up an error dialog and call the \"Exit\" message."
                n144 = call-poly <vilib>:"Delacor_lib_QMH_Enqueue Message (poly).vi"("Priority Message? (F)"=TRUE, "Message"="Exit", "Message Queue in"=w333) -> ("error out"=w334:errorcluster)  [unwired: 7 in, 1 out]
              }
              frame True {
                # "If the module was launched externally, calling the Error Reported broadcast VI is the only action performed by the \"Error\" message. The module's caller can then process the error appropriately."
              }
            }
            n145 = Merge Errors(w326, w325) -> (w321:errorcluster)
            n146 = local write "error out"(w321) -> ()
          }
          frame "Confirm Quit" {
            # "#CodeNeeded - If you want to provide an \"Are you sure\" dialog (or some other notification) before the application exits, place that code here. This message is typically sent from a Panel Close? event."
            # "Confirm Quit - Message that can confirm whether or not the user wants to exit the application."
            n147 = call-poly <vilib>:"Delacor_lib_QMH_Enqueue Message (poly).vi"("Priority Message? (F)"=TRUE, "error in"=w341, "Message"="Exit", "Message Queue in"=w337) -> ("error out"=w338:errorcluster)  [unwired: 6 in, 1 out]
            n148 = Merge Errors(w338) -> (w339:errorcluster)
          }
          frame "Exit" {
            w348 = 91  # 91: not all Exit messages will have an argument
            w353 = TRUE  # Stop the VI
            # "Release the message queue reference"
            # "Exit - Exit the application."
            n149 = Variant To Data(error in=w356, type=T5 {"Origin"="", "Exit via Stop Module Req?"=FALSE, "Wait for Module to stop?"=FALSE} ("Stop Argument"), Variant=w350) -> (data=w346:T5, error out=w349:errorcluster)
            n150 = call <vilib>:"Clear Errors.vi"("error in (no error)"=w349, "specific error code to clear (0: all)"=w348) -> ("error out"=w355:errorcluster)  [unwired: 4 in, 1 out]
            n151 = control-ref of="This VI"() -> (w344:refnum<vi>)
            n152 = call-dynamic "Delacor_lib_QMH_Release Message Queue.vi"("error in"=w355, "Message Queue"=w354) -> ("error out"=w352:errorcluster)  [unwired: 9 in]
            n153 = call "Handle Exit.vi"("Stop Argument"=w346, "Admin in"=w343, "VI reference"=w344) -> ("error out"=w345:errorcluster)  [unwired: 7 in, 1 out]
            n154 = Merge Errors(w345, w352) -> (w351:errorcluster)
            n155 = call "Error Reported.vi"("Error"=w351) -> ()  [unwired: 10 in, 1 out]
          }
          frame Default {
            # "'Default' case only runs if there is a message that isn't defined in any of the other cases.  Output a programming error."
            n156 = call "Module Name--constant.vi"() -> ("Module Name"=w357:string)  [unwired: 11 in]
            n157 = xnode "Error Ring"("parameter 0"=w358, "parameter 1"=w357) -> ("error out"=w359:errorcluster)
          }
        }
        n158 = call-dynamic "Delacor_lib_QMH_Error Handler - Message Handling Loop.vi"("error in"=w177, "Message Queue in"=w168) -> ("dup error in"=w167:errorcluster)  [unwired: 8 in, 1 out]
      }
    }
    frame Error {
      # "Synchronize Caller Events.vi will inform Start Module.vi that the module has launched and will let the code calling Start Module.vi register for broadcasts and would permit the caller receive the broadcast that an error occurred at launch time."
      n159 = call "Synchronize Caller Events.vi"("Singleton Module Admin in"=w373) -> ("error out"=w370:errorcluster)  [unwired: 9 in, 1 out]
      n160 = call-dynamic "Delacor_lib_QMH_Release Message Queue.vi"("Message Queue"=w369) -> ()  [unwired: 10 in, 1 out]
      n161 = call "Module Name--constant.vi"() -> ("Module Name"=w376:string)  [unwired: 11 in]
      n162 = Format Into String(format string="An error occurred during initialization. %s is no longer running.", w376) -> (resulting string=w374:string)  [unwired: 2 in, 1 out]
      n163 = Merge Errors(w372, w370) -> (w371:errorcluster)
      n164 = call "Error Reported.vi"("Additional Information"=w374, "Error"=w371) -> ()  [unwired: 9 in, 1 out]
    }
  }
  n165 = Merge Errors(w15, w23) -> (w14:errorcluster)
  n166 = call "Close Module.vi"("error in (no error)"=w14, "Module Admin in"=w24) -> ("error out"=w17:errorcluster, "External Launch"=w13:bool, "Module Admin out"=w16:refnum<class "Delacor_lib_QMH_Module Admin.lvclass">)  [unwired: 7 in]
  n167 = Unregister For Events(event registration refnum=w22, error in=w17) -> (error out=w7:errorcluster)
  "error out" <- w7
  n168 = case "External Launch?" shown="True" w13 {
    tunnel: w7 -> [_ w378]
    frame False {
    }
    frame True {
      n169 = case shown="No Error" w378 {
        frame No Error {
          n170 = invoke class="VI" method="FP.Close"() -> ()  [unwired: 3 in, 3 out]
        }
        frame Error {
          n171 = invoke class="VI" method="FP.Open"("Activate"=TRUE ("Activate?")) -> ()  [unwired: 4 in, 5 out]
        }
      }
    }
  }
  n172 = local write "Module Admin"(w16) -> ()
  n173 = call "Module Name--constant.vi"() -> ("Module Name"=w6:string)  [unwired: 11 in]
  n174 = Format Into String(format string="Module %s stopped", w6) -> (resulting string=w8:string)  [unwired: 2 in, 1 out]
  n175 = call <vilib>:"INFO.vi"("Message"=w8, "error in"=w7) -> ()  [unwired: 9 in, 1 out]
